vi "1D Interpolated Table Lookup.vi"(8 "Min Range":dbl format="%#_13g", 9 "Max Range":dbl=100.0 format="%#_13g", 10 "1d Accell Downshift Input Table":bool[](array[boolean]), 11 "Input":dbl=20.0 format="%#_13g") -> (3 "Shift?":bool)   [LabVIEW 2013]
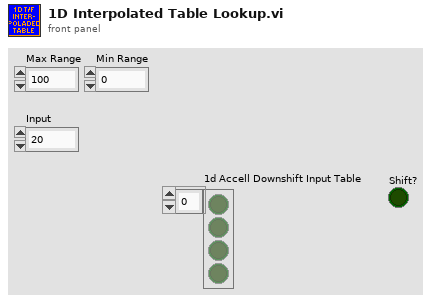
[diagram p1: front panel]
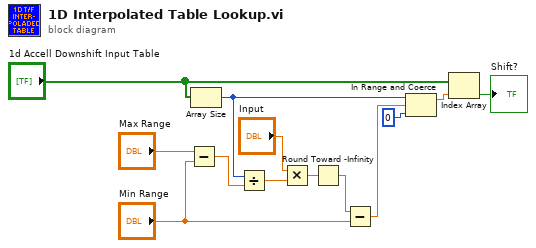
[diagram p0: block diagram]
diagram:
  n1 = Subtract(x="Max Range", y="Min Range") -> (x-y=w8:dbl)
  n2 = Array Size(array="1d Accell Downshift Input Table") -> (size(s)=w6:i32)
  n3 = Divide(x=w6, y=w8) -> (x/y=w10:dbl)
  n4 = Multiply(x="Input", y=w10) -> (x*y=w9:dbl)
  n5 = Round Toward -Infinity(1:w9) -> (0:w3:dbl)
  n6 = Subtract(x=w3, y="Min Range") -> (x-y=w1:dbl)
  n7 = In Range and Coerce(upper limit=w6, x=w1, lower limit=0) -> (coerced(x)=w4:dbl)  [unwired: 1 out]
  n8 = Index Array(array="1d Accell Downshift Input Table", index=w4) -> (element=→"Shift?":bool)
